vi "Tag_Size.vi"(8 "error in (no error)":errorcluster, 11 "tag handle":i32) -> (0 "error out":errorcluster, 2 "tag size":i32, 3 "tag handle out":i32)   [LabVIEW 2016]
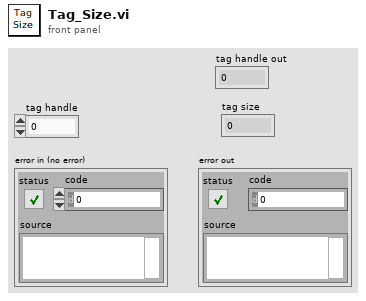
[diagram p1: front panel]
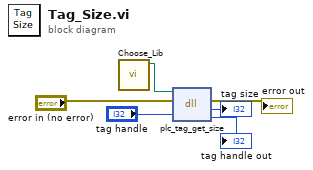
[diagram p0: block diagram]
diagram:
  n1 = call "Choose_Lib.vi"() -> ("appended path"=w1:path)  [unwired: 11 in]
  n2 = dll-call lib="home/dbowden/Desktop/libplctag-master/build/bin_dist/libplctag.so" fn="plc_tag_get_size"(path in=w1, error in="error in (no error)", "tag"="tag handle") -> (error out=→"error out":errorcluster, "return type"=→"tag size":i32, "tag"=→"tag handle out":i32)  [unwired: 1 in, 1 out]
